vi "Read JSON Config.vi"(8 "error in (no error)":errorcluster, 10 "JSON Config":string, 11 "Const_WFM in":refnum<class "Const_WFM.lvclass">) -> (0 "error out":errorcluster, 3 "Const_WFM out":refnum<class "Const_WFM.lvclass">)   [LabVIEW 2021, in "Const_WFM.lvclass"]
uses:
  Const_WFM.lvclass
  C:/Program Files (x86)/National Instruments/LabVIEW 2021/vi.lib/TSA/Abstract Data Classes/Abs_Types/Type/Abs_Type.lvclass
  Const_WFM.lvclass/Const_WFM.ctl
  48dc8292-d18f-4e5c-9842-eb0e28dfcac3.vi
  <vilib>/JDP Science/JSONtext/Find Item.vi
  <vilib>/JDP Science/JSONtext/Next JSON Value.vi
  <vilib>/JDP Science/JSONtext/String Subset.vi
  <vilib>/JDP Science/JSONtext/Parsing/Advance past next JSON Value (inlined COPY).vi
  <vilib>/JDP Science/JSONtext/Parsing/Advance past whitespace.vi
  <vilib>/JDP Science/JSONtext/Parsing/Advance past String.vi
  <vilib>/JDP Science/JSONtext/Parsing/Advance past Number.vi
  <vilib>/JDP Science/JSONtext/Parsing/Advance past Line Ending.vi
  <vilib>/Utility/LVClass/Get LV Class Name.vi
  <vilib>/JDP Science/JSONtext/Parsing/Parse Full Path or Item Name.vi
  <vilib>/JDP Science/JSONtext/Parsing/Advance past Array.vi
  <vilib>/JDP Science/JSONtext/Parsing/Advance past Object.vi
  <vilib>/JDP Science/JSONtext/support/Error Cluster From Code.vi
  <vilib>/JDP Science/JSONtext/Offset/Find Item Locations by Path.vi
  <vilib>/JDP Science/JSONtext/JSON text to Variant.vi
  <vilib>/JDP Science/JSONtext/LVClass Serializer/JSONtext LVClass Serializer.lvclass
  Abs_Types/Waveform/Abs_Waveform.lvclass
  Abs_Types/Type/Abs_Type.lvclass
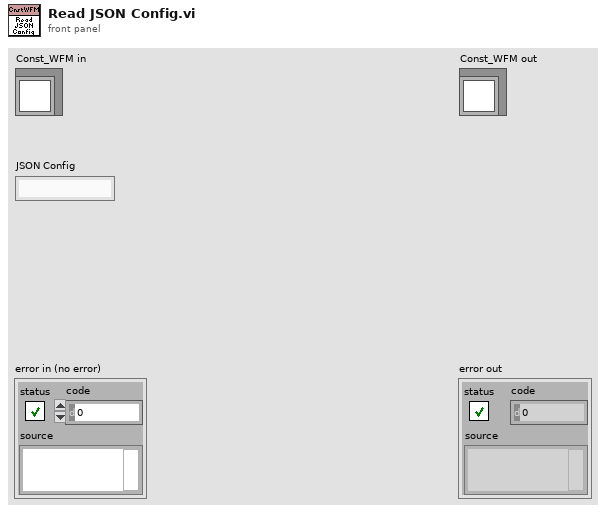
[diagram p1: front panel]
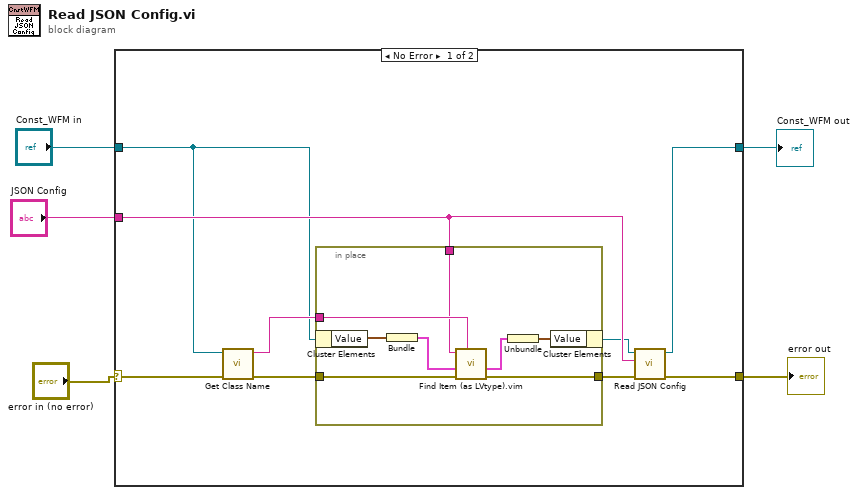
[diagram p0: block diagram]
diagram:
  n1 = case shown="No Error" "error in (no error)" {
    selector: "error in (no error)" -> [w11 w23]
    tunnel: [w14 w23] -> w4
    tunnel: [w13 w24] -> w2
    tunnel: "JSON Config" -> [w8 _]
    tunnel: "Const_WFM in" -> [w7 w24]
    frame No Error {
      n2 = call "Get Class Name.vi"("error in (no error)"=w11, "Abs_Type in"=w7) -> ("error out"=w9:errorcluster, "class name"=w10:string)  [unwired: 8 in]
      n3 = in-place {
        in-place-border: [w20] -> w12
        in-place-border: w10 -> [w19]
        in-place-border: w9 -> [w18]
        in-place-border: w8 -> [w17]
        n4 = in-place-cluster #1(w7) -> ("Value"=w16:waveform(dbl))
        n5 = Bundle("Value"=w16) -> (w21:cluster{"Value":waveform(dbl)})  [unwired: 1 in]
        n6 = call "Find Item (as LVtype).vim"("$Path or Item Name"=w19, "error in (no error)"=w18, "Data Type and Default Value"=w21, "JSON"=w17) -> ("error out"=w20:errorcluster, "Data"=w22:cluster{"Value":waveform(dbl)})  [unwired: 4 in, 2 out]
        n7 = Unbundle(w22) -> ("Value"=w15:waveform(dbl))
        n8 = in-place-cluster #1("Value"=w15) -> (w6:refnum<class "Const_WFM.lvclass">)
      }
      n9 = call-parent "Read JSON Config.vi"("error in (no error)"=w12, "JSON Config"=w8, "Abs_Type in"=w6) -> ("error out"=w14:errorcluster, "Abs_Type out"=w13:refnum<class "Const_WFM.lvclass">)  [unwired: 7 in]
    }
    frame Error {
    }
  }
  "error out" <- w4
  "Const_WFM out" <- w2
